vi "GetGoalPos.vi"(0 "Image":T1, 1 "error in":errorcluster) -> (2 "Number of Particles (Particle Analysis 1)":i32, 3 "Particle Measurements (Pixels)":dbl[][](array[numeric]) format="%.2f", 4 "error out":errorcluster)   [LabVIEW 2015]
uses:
  <vilib>/vision/Image Controls.llb/IMAQ Image.ctl
  <vilib>/vision/NI_Vision_Development_Module.lvlib
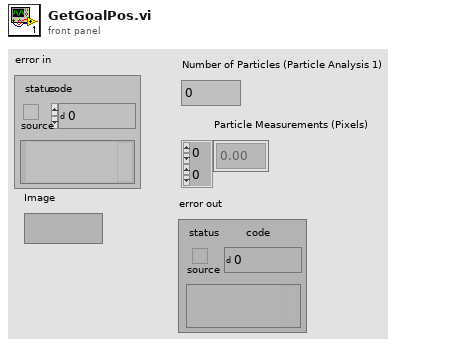
[diagram p1: front panel]
types:
  T1 = typedef "IMAQ Image.ctl" = refnum<image>
  T2 = typedef "Particle Parameters" = i32
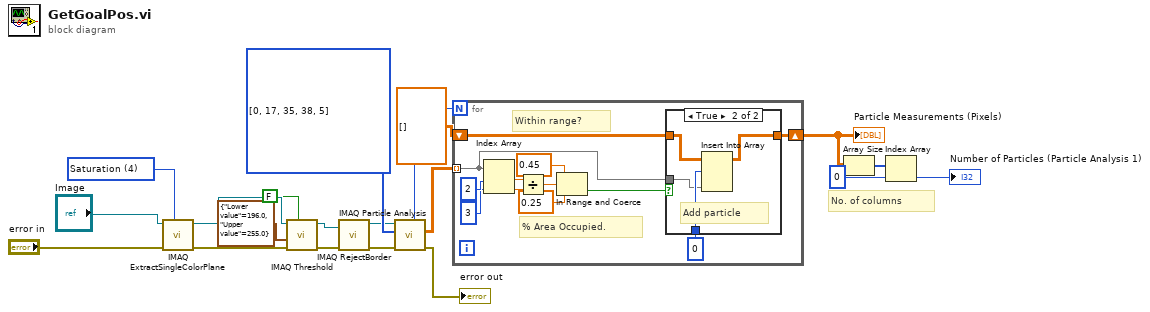
[diagram p0: block diagram]
diagram:
  w15 = T2[] [0, 17, 35, 38, 5] items=["Center of Mass X", "Center of Mass Y", "First Pixel X", "First Pixel Y", "Bounding Rect Left", "Bounding Rect Top", "Bounding Rect Right", "Bounding Rect Bottom", "Max Feret Diameter Start X", "Max Feret Diameter Start Y", "Max Feret Diameter End X", "Max Feret Diameter End Y", "Max Horiz. Segment Length Left", "Max Horiz. Segment Length Right", "Max Horiz. Segment Length Row", "-", "Bounding Rect Width", "Bounding Rect Height", "Bounding Rect Diagonal", "Perimeter", "Convex Hull Perimeter", "Holes' Perimeter", "Max Feret Diameter", "Equivalent Ellipse Major Axis", "Equivalent Ellipse Minor Axis", "Equivalent Ellipse Minor Axis (Feret)", "Equivalent Rect Long Side", "Equivalent Rect Short Side", "Equivalent Rect Diagonal", "Equivalent Rect Short Side (Feret)", "Average Horiz. Segment Length", "Average Vert. Segment Length", "Hydraulic Radius", "Waddel Disk Diameter", "-", "Area", "Holes' Area", "Particle & Holes' Area", "Convex Hull Area", "Image Area", "-", "Number of Holes", "Number of Horiz. Segments", "Number of Vert. Segments", "-", "Orientation", "Max Feret Diameter Orientation", "-", "% Area/Image Area", "% Area/(Particle & Holes' Area)", "Ratio of Equivalent Ellipse Axes", "Ratio of Equivalent Rect Sides", "-", "Elongation Factor", "Compactness Factor", "Heywood Circularity Factor", "Type Factor", "-", "Sum X", "Sum Y", "Sum XX", "Sum XY", "Sum YY", "Sum XXX", "Sum XXY", "Sum XYY", "Sum YYY", "-", "Moment of Inertia XX", "Moment of Inertia XY", "Moment of Inertia YY", "Moment of Inertia XXX", "Moment of Inertia XXY", "Moment of Inertia XYY", "Moment of Inertia YYY", "Norm. Moment of Inertia XX", "Norm. Moment of Inertia XY", "Norm. Moment of Inertia YY", "Norm. Moment of Inertia XXX", "Norm. Moment of Inertia XXY", "Norm. Moment of Inertia XYY", "Norm. Moment of Inertia YYY", "Hu Moment 1", "Hu Moment 2", "Hu Moment 3", "Hu Moment 4", "Hu Moment 5", "Hu Moment 6", "Hu Moment 7"] ("Pixel Measurements")
  w20 = 4 items=["Red", "Green", "Blue", "Hue", "Saturation", "Luminance", "Value", "Intensity"] ("Color Plane")
  # "No. of columns"
  n1 = call "IMAQ ExtractSingleColorPlane"("Color Plane"=w20, "error in (no error)"="error in", "Image Src"="Image") -> ("error out"=w17:errorcluster, "Image Dst Out"=w18:T1)  [unwired: 1 in, 6 out]
  n2 = call "IMAQ Threshold"("Keep/Replace Value (Replace)"=FALSE, "error in (no error)"=w17, "Range"=cluster{"Lower value":sgl, "Upper value":sgl} {"Lower value"=196.0, "Upper value"=255.0}, "Image Src"=w18) -> ("error out"=w4:errorcluster, "Image Dst Out"=w3:T1)  [unwired: 2 in, 4 out]
  n3 = call "IMAQ RejectBorder"("error in (no error)"=w4, "Image Src"=w3) -> ("error out"=w1:errorcluster, "Image Dst Out"=w2:T1)  [unwired: 4 in]
  n4 = call "IMAQ Particle Analysis"("error in (no error)"=w1, "Pixel Measurements"=w15, "Image"=w2) -> ("error out"=→"error out":errorcluster, "Particle Measurements (Pixels)"=w14:dbl[][], "Number of Particles"=w11:i32)  [unwired: 2 in, 4 out]
  n5 = for {
    N: w11 -> [_]
    tunnel: w14 -> [w23] mode=indexing
    shift-right: [w24] -> w10
    shift-left: dbl[][] [] -> [w25]
    # "Within range?"
    # "% Area Occupied."
    n6 = Index Array(array=w23, index #1=2 ("index"), index #2=3 ("index")) -> (element #1=w29:dbl, element #2=w30:dbl)
    n7 = Divide(x=w29, y=w30) -> (x/y=w28:dbl)
    n8 = In Range and Coerce(upper limit=0.45, x=w28, lower limit=0.25) -> (In Range?=w22:bool)  [unwired: 1 out]
    n9 = case shown="True" w22 {
      tunnel: w25 -> [w33 w35]
      tunnel: [w33 w34] -> w24
      tunnel: 0 -> [_ w37]
      tunnel: w23 -> [_ w36]
      frame False {
        # "Do not add\nparticle"
      }
      frame True {
        # "Add particle"
        n10 = Insert Into Array(array=w35, index (row)=w37, new element=w36) -> (w34:dbl[][])  [unwired: 1 in]
      }
    }
  }
  "Particle Measurements (Pixels)" <- w10
  n11 = Array Size(array=w10) -> (size(s)=w9:i32[])
  n12 = Index Array(array=w9, index=0) -> (element=→"Number of Particles (Particle Analysis 1)":i32)
